vi "Tunnel.vi"() -> ()   [LabVIEW 2022 SP3]
panel:
  out "Number of Iterations":dbl
  out "Current number":dbl format="%#.0f"
  in  "Number to match":dbl min=0.0 max=1000.0 step=1.0
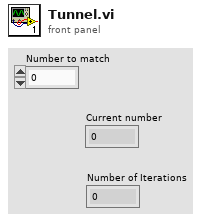
[diagram p1: front panel]
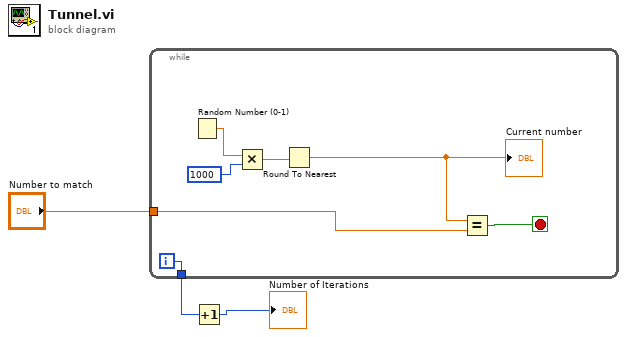
[diagram p0: block diagram]
diagram:
  n1 = while {
    tunnel: "Number to match" -> [w7]
    tunnel: [w5] -> w2
    i -> [w5]
    stop <- w6 stop-if-true
    n2 = Random Number (0-1)() -> (number: 0 to 1=w10:dbl)
    n3 = Multiply(x=w10, y=1000) -> (x*y=w8:dbl)
    n4 = Round To Nearest(number=w8) -> (nearest integer value=w4:dbl)
    "Current number" <- w4
    n5 = Equal?(x=w4, y=w7) -> (x = y?=w6:bool)
  }
  n6 = Increment(x=w2) -> (x+1=→"Number of Iterations":i32)
